vi "Array2ini.vi"(1 "数组":T1[](array[typedef]), 2 "路径":path) -> ()   [LabVIEW 2019]
uses:
  ctl/InfoOfPlayer.ctl
  <vilib>/Utility/config.llb/NI_LVConfig.lvlib
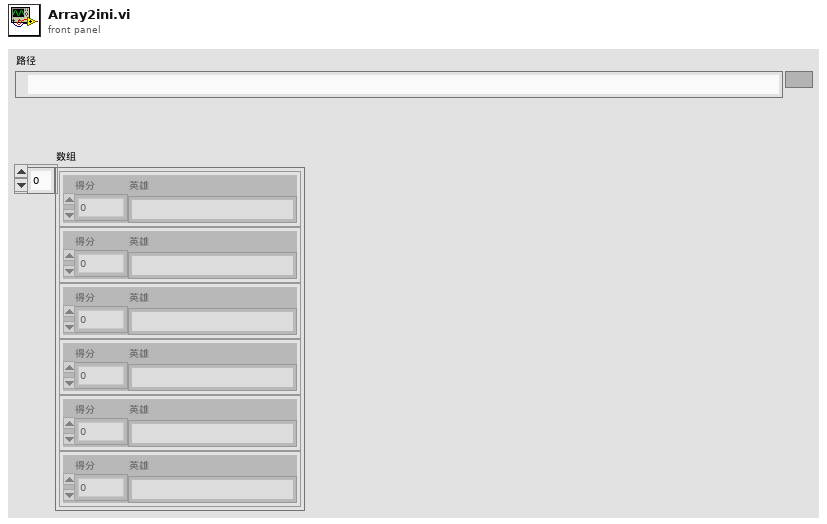
[diagram p1: front panel]
types:
  T1 = typedef "InfoOfPlayer.ctl" = cluster{"得分":i32, "英雄":string}
  T2 = typedef "NI_LVConfig.lvlib/Config Data RefNum.ctl" = refnum<k1>
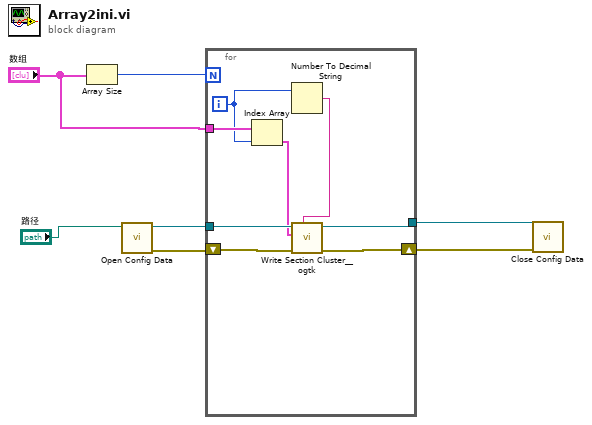
[diagram p0: block diagram]
diagram:
  n1 = Array Size(array="数组") -> (size(s)=w7:i32)
  n2 = call <vilib>:"Open Config Data.vi"("configuration file path"="路径") -> ("error out"=w4:errorcluster, "refnum"=w5:T2)  [unwired: 8 in, 1 out]
  n3 = for {
    N: w7 -> [_]
    tunnel: w5 -> [w15]
    shift-right: [w13] -> w3
    shift-left: w4 -> [w14]
    tunnel: [w12] -> w2
    tunnel: "数组" -> [w11]
    i -> [w10]
    n4 = Index Array(array=w11, index=w10) -> (element=w8:T1)
    n5 = Number To Decimal String(number=w10) -> (decimal integer string=w9:string)  [unwired: 1 in]
    n6 = call <userlib>:"Write Section Cluster__ogtk.vi"("section (optional)"=w9, "error in (no error)"=w14, "Section Formatted Cluster"=w8, "refnum"=w15) -> ("error out"=w13:errorcluster, "dup refnum"=w12:T2)  [unwired: 6 in]
  }
  n7 = call <vilib>:"Close Config Data.vi"("error in (no error)"=w3, "refnum"=w2) -> ()  [unwired: 8 in, 2 out]
